vi "AddSysPath.vi"(8 "错误输入":errorcluster, 11 "Path":string) -> (0 "error out":errorcluster caption="错误输出", 3 "success?":bool)   [LabVIEW 2018, in "Win32API.lvlib"]
uses:
  Win32API.lvlib
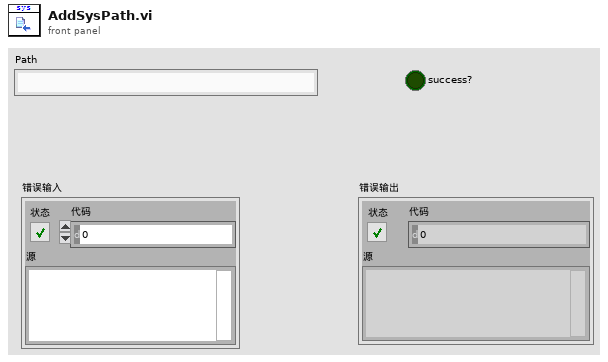
[diagram p1: front panel]
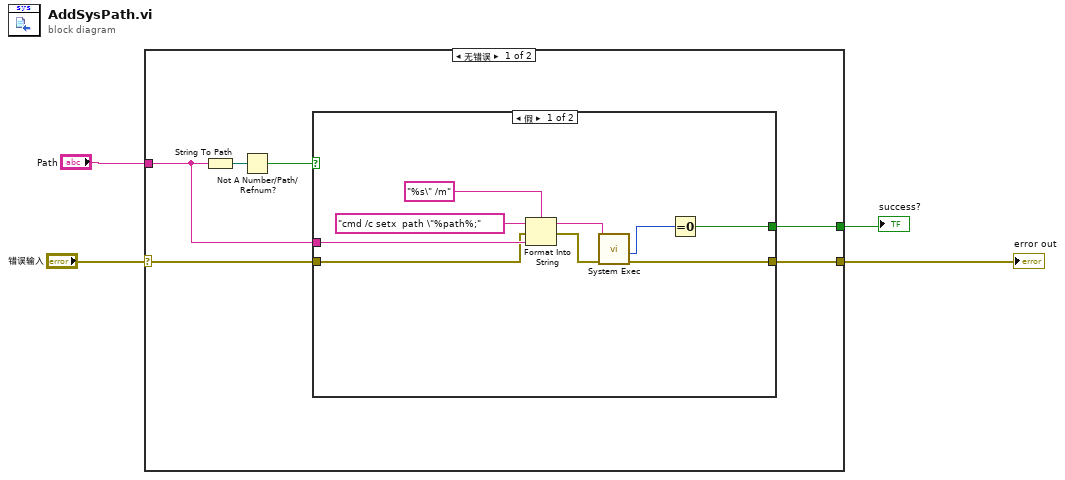
[diagram p0: block diagram]
diagram:
  n1 = case shown="无错误" "错误输入" {
    selector: "错误输入" -> [w9 w21]
    tunnel: [w10 w21] -> w4
    tunnel: "Path" -> [w6 _]
    tunnel: [w5 _] -> w1
    frame No Error {
      n2 = String To Path(string=w6) -> (path=w8:path)
      n3 = Not A Number/Path/Refnum?(number/path/refnum=w8) -> (NaN/Path/Refnum?=w7:bool)
      n4 = case shown="假" w7 {
        tunnel: w6 -> [w17 _]
        tunnel: [w15 w20] -> w10
        tunnel: w9 -> [w14 w20]
        tunnel: [w12 _] -> w5
        frame False {
          n5 = Format Into String(format string="%s\" /m" ("command line"), initial string="cmd /c setx  path \"%path%;" ("初始字符串"), error in=w14, w17) -> (resulting string=w11:string, error out=w16:errorcluster)
          n6 = call <vilib>:"System Exec.vi"("error in (no error)"=w16, "command line"=w11) -> ("error out"=w15:errorcluster, "return code"=w13:i32)  [unwired: 6 in, 2 out]
          n7 = Equal To 0?(x=w13) -> (x = 0?=w12:bool)
        }
        frame True {
        }
      }
    }
    frame Error {
    }
  }
  "error out" <- w4
  "success?" <- w1
